vi "ziGetCurrentCalcVal.vi"(4 "Gain (), Shunt (ohm)":dbl, 5 "VGain":i32, 6 "Imp50 (F)":bool, 7 "R":dbl, 10 "Voltage (Vrms)":cdb format="%#_6p", 11 "Mode":T1(ring)) -> (2 "I (Arms)":cdb format="%#_6p")   [LabVIEW 2009, in "Zurich Instruments LabOne.lvlib"]
uses:
  <instrlib>/Zurich Instruments LabOne/Zurich Instruments LabOne.lvlib
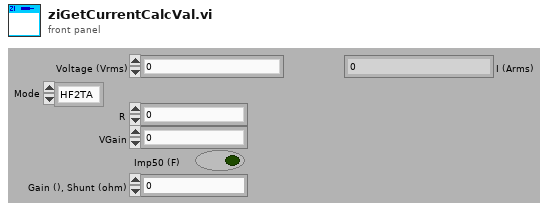
[diagram p1: front panel]
types:
  T1 = enum16{"HF2TA", "HF2CA", "Int. Shunt", "Ext. Shunt"}
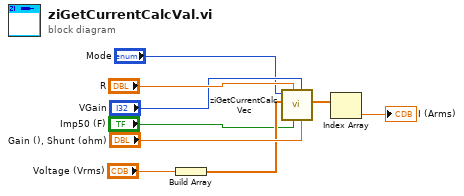
[diagram p0: block diagram]
diagram:
  n1 = Build Array("Voltage (Vrms)") -> (w4:cdb[])
  n2 = call <instrlib>:"ziGetCurrentCalcVec.vi"("Gain (), Shunt (ohm)"="Gain (), Shunt (ohm)", "VGain"="VGain", "Imp50 (F)"="Imp50 (F)", "R"="R", "DemodVoltage (Vrms)"=w4, "Mode"="Mode") -> ("I (Arms)"=w5:cdb[])  [unwired: 5 in]
  n3 = Index Array(array=w5) -> (element=→"I (Arms)":cdb)  [unwired: 1 in]
